vi "Check Steering Input.vi"(8 "error in (no error)":errorcluster, 11 "RDS Local Remote Actor in":refnum<class "RDS Local Remote Actor.lvclass">) -> (0 "error out":errorcluster, 3 "RDS Local Remote Actor out":refnum<class "RDS Local Remote Actor.lvclass">)   [LabVIEW 2015, in "RDS Local Remote Actor.lvlib" / "RDS Local Remote Actor.lvclass"]
uses:
  RDS Local Remote Actor.lvclass
  RDS Local Remote Actor.lvclass/RDS Local Remote Actor.ctl
  Libraries/RDS Child Messages/Helm/Steering Command/Steering Command Cntrl.ctl
  Libraries/RDS Child Messages/RDS Child Messages.lvlib
  Libraries/Geo/RDS Libraries.lvlib
  RDS Helm Actor/RDS Helm Actor.lvlib
  RDS Parent Actor/RDS Parent Actor/RDS Parent Actor.lvclass
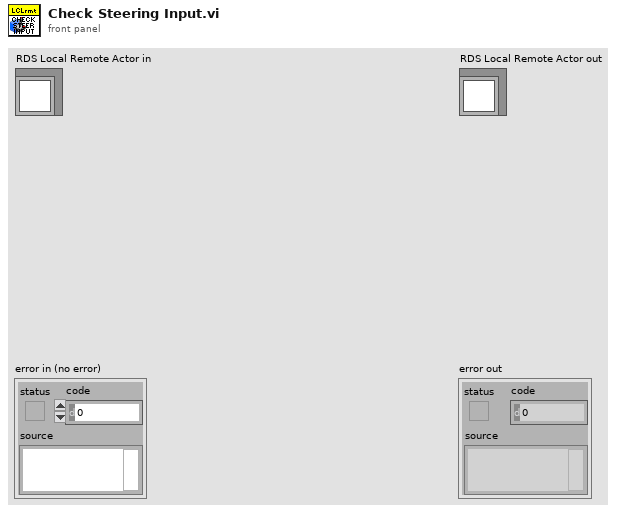
[diagram p1: front panel]
types:
  T1 = typedef "RDS Child Messages.lvlib/Steering Command Cntrl.ctl" = cluster{"Throttle":i16, "Rudder":i8, "Duration (s)":u16}
  T2 = cluster{"axis info":cluster{"X axis":i32, "Y axis":i32, "Z axis":i32, "X axis rotation":i32, "Y axis rotation":i32, "Z axis rotation":i32, "U axis":i32, "V axis":i32}, "button info":cluster{"button 1":bool, "button 2":bool, "button 3":bool, "button 4":bool, "button 5":bool, "button 6":bool, "button 7":bool, "button 8":bool, "button 9":bool, "button 10":bool, "button 11":bool, "button 12":bool, "button 13":bool, "button 14":bool, "button 15":bool, "button 16":bool, "button 17":bool, "button 18":bool, "button 19":bool, "button 20":bool, "button 21":bool, "button 22":bool, "button 23":bool, "button 24":bool, "button 25":bool, "button 26":bool, "button 27":bool, "button 28":bool, "button 29":bool, "button 30":bool, "button 31":bool, "button 32":bool}, "direction info":cluster{"pov 1":i32, "pov 2":i32, "pov 3":i32, "pov 4":i32}}
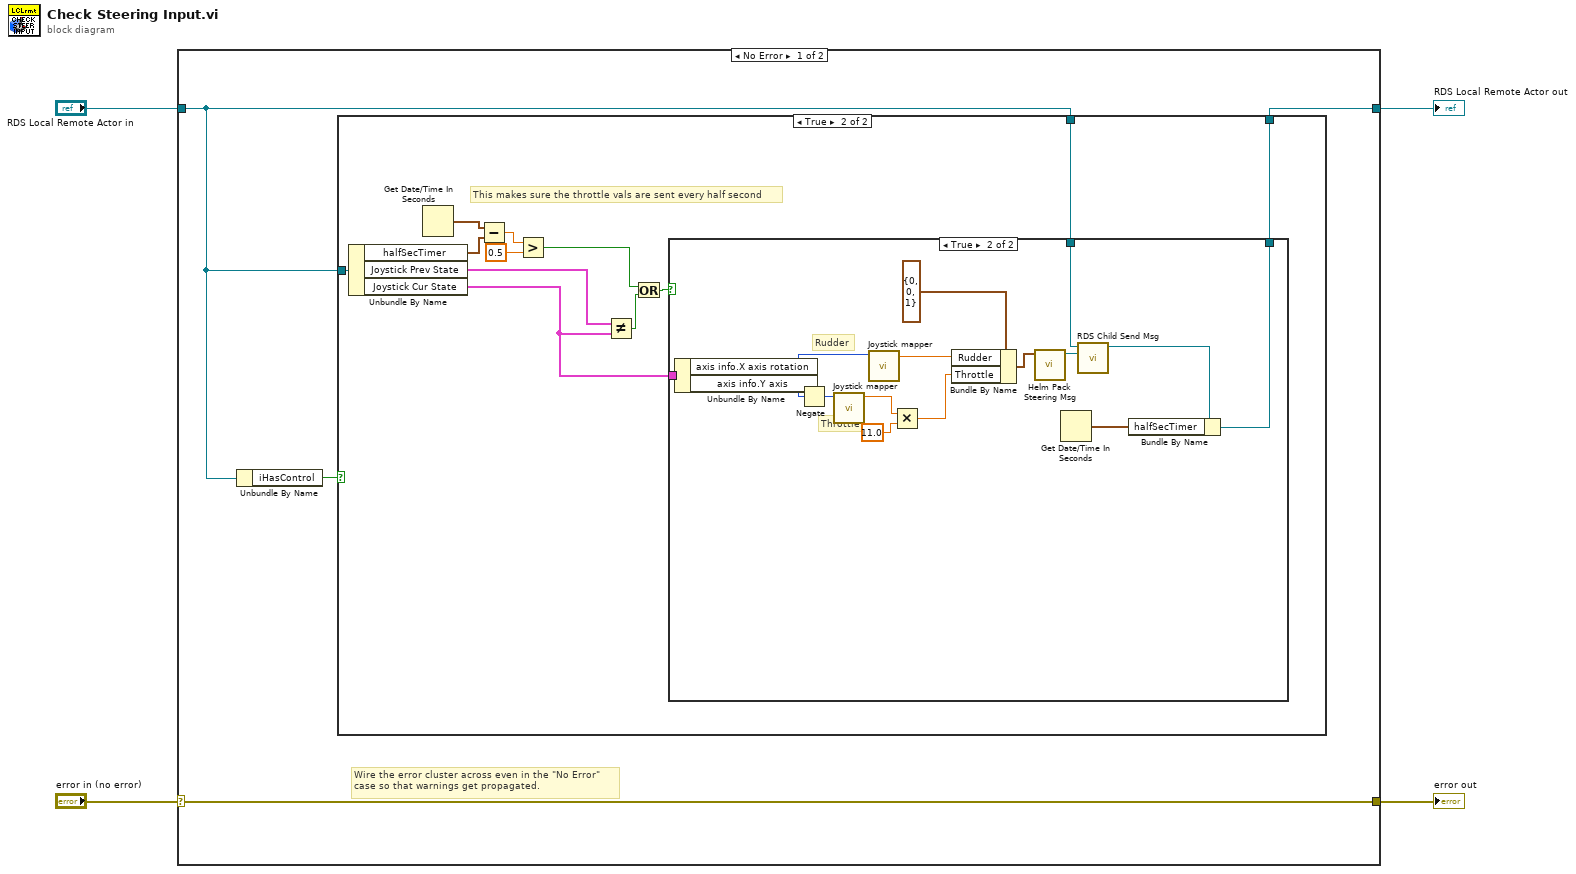
[diagram p0: block diagram]
diagram:
  n1 = case shown="No Error" "error in (no error)" {
    selector: "error in (no error)" -> [w8 w39]
    tunnel: [w8 w39] -> w3
    tunnel: [w5 w38] -> w1
    tunnel: "RDS Local Remote Actor in" -> [w6 w38]
    frame No Error {
      # "Wire the error cluster across even in the \"No Error\"\ncase so that warnings get propagated."
      n2 = Unbundle By Name(w6) -> ("iHasControl"=w7:bool)
      n3 = case shown="True" w7 {
        tunnel: w6 -> [_ w21]
        tunnel: w6 -> [w9 w12]
        tunnel: [w9 w10] -> w5
        frame False {
        }
        frame True {
          # "This makes sure the throttle vals are sent every half second"
          n4 = Unbundle By Name(w21) -> ("halfSecTimer"=w19:timestamp, "Joystick Prev State"=w20:T2, "Joystick Cur State"=w11:T2)
          n5 = Get Date/Time In Seconds() -> (seconds since 1Jan1904=w18:timestamp)
          n6 = Subtract(x=w18, y=w19) -> (x-y=w17:dbl)
          n7 = Greater?(x=w17, y=0.5) -> (0:w15:bool)
          n8 = Not Equal?(x=w20, y=w11) -> (x != y?=w14:bool)
          n9 = Or(x=w15, y=w14) -> (x .or. y?=w13:bool)
          n10 = case shown="True" w13 {
            tunnel: w11 -> [_ w37]
            tunnel: w12 -> [w22 w30]
            tunnel: [w22 w26] -> w10
            frame False {
            }
            frame True {
              # "Throttle"
              # "Rudder"
              n11 = Unbundle By Name(w37) -> ("axis info.X axis rotation"=w36:i32, "axis info.Y axis"=w35:i32)
              n12 = Negate(x=w35) -> (-x=w34:i32)
              n13 = call "Joystick mapper.vi"("Input"=w34) -> ("Output"=w24:dbl)  [unwired: 10 in]
              n14 = call "Joystick mapper.vi"("Input"=w36) -> ("Output"=w33:dbl)  [unwired: 10 in]
              n15 = Multiply(x=w24, y=11.0) -> (x*y=w23:dbl)
              n16 = Bundle By Name(cluster=T1 {"Throttle"=0, "Rudder"=0, "Duration (s)"=1} ("Steering Command Control"), "Rudder"=w33, "Throttle"=w23) -> (w31:T1)
              n17 = call "Helm Pack Steering Msg.vi"("Steering Command Control"=w31) -> ("Steer Msg"=w29:refnum<class "Steering Command.lvclass">)  [unwired: 9 in, 1 out]
              n18 = Get Date/Time In Seconds() -> (seconds since 1Jan1904=w27:timestamp)
              n19 = call "RDS Child Send Msg.vi"("RDS Message"=w29, "RDS Parent Actor in"=w30) -> ("RDS Parent Actor out"=w28:refnum<class "RDS Local Remote Actor.lvclass">)  [unwired: 8 in, 1 out]
              n20 = Bundle By Name(cluster=w28, "halfSecTimer"=w27) -> (w26:refnum<class "RDS Local Remote Actor.lvclass">)
            }
          }
        }
      }
    }
    frame Error {
    }
  }
  "error out" <- w3
  "RDS Local Remote Actor out" <- w1
